vi "FPGA_SPI_ReadAuto.vi"(8 "error in (no error)":errorcluster, 9 "Bytes per Sample":u32, 10 "Samples to Read":u32) -> (0 "error out":errorcluster, 2 "Data":u8[][](array[numeric]))   [LabVIEW 2017]
uses:
  <vilib>/Utility/error.llb/Error Cluster From Error Code.vi
  <vilib>/rvi/errors/niLvFpgaAdjustHostInterfaceError.vi
  <vilib>/rvi/interface/nirviMethod/nirviMethod.xnode
  <vilib>/Rock Robotics/SystemInterfaces/System/FPGA_SystemFRC FPGA Ref.ctl
  <vilib>/FPGAPlugInAG/Dynamic/niLvFpga_ReadFifo_Dynamic.vi
  <vilib>/rvi/errors/niLvFpgaMergeErrorWithErrorCode.vi
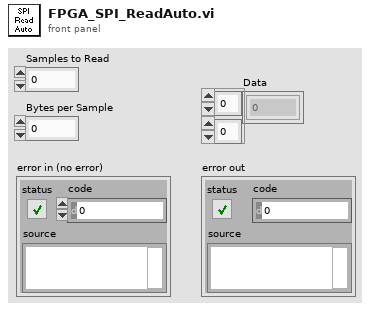
[diagram p1: front panel]
types:
  T1 = typedef "FPGA_SystemFRC FPGA Ref.ctl" = refnum<k20>
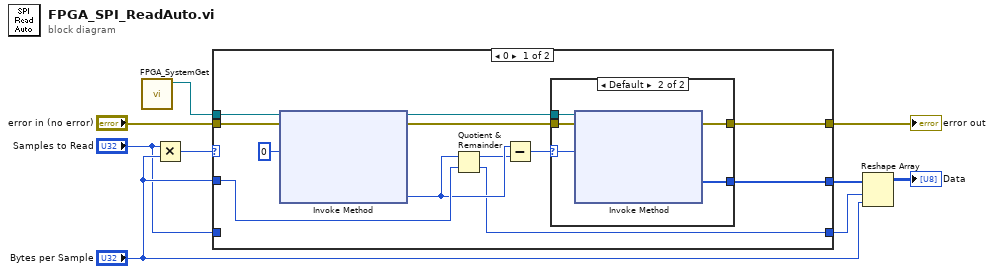
[diagram p0: block diagram]
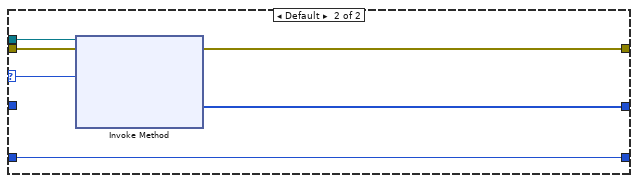
[diagram p3: hidden frame]
diagram:
  n1 = call <vilib>:"FPGA_SystemGet.vi"() -> ("FRC FPGA Ref"=w7:T1)  [unwired: 11 in]
  n2 = Multiply(x="Samples to Read", y="Bytes per Sample") -> (x*y=w5:u32)
  n3 = case shown="0" w5 {
    selector: w5 -> [_ w30]
    tunnel: [w16 w33] -> w9
    tunnel: "error in (no error)" -> [w21 w32]
    tunnel: w7 -> [w20 w31]
    tunnel: [w19 w29] -> w4
    tunnel: "Bytes per Sample" -> [w15 _]
    tunnel: [w10 w28] -> w1
    tunnel: "Samples to Read" -> [_ w28]
    frame 0 {
      n4 = xnode "Invoke Method"("FPGA VI Reference In"=w20, "error in"=w21, "Number of Elements"=u32 0) -> ("FPGA VI Reference Out"=w18:T1, "error out"=w17:errorcluster, "Elements Remaining"=w14:u32)  [unwired: 1 in, 1 out]
      n5 = Quotient & Remainder(x=w14, y=w15) -> (x-y*floor(x/y)=w13:u32, floor(x/y)=w10:u32)
      n6 = Subtract(x=w14, y=w13) -> (x-y=w12:u32)
      n7 = case shown="Default" w12 {
        selector: w12 -> [_ w24]
        tunnel: [_ w23] -> w19
        tunnel: w18 -> [_ w27]
        tunnel: w17 -> [w22 w26]
        tunnel: [w22 w25] -> w16
        frame 0 {
        }
        frame Default {
          n8 = xnode "Invoke Method"("FPGA VI Reference In"=w27, "error in"=w26, "Number of Elements"=w24) -> ("error out"=w25:errorcluster, "Data"=w23:u8[])  [unwired: 1 in, 2 out]
        }
      }
    }
    frame Default {
      n9 = xnode "Invoke Method"("FPGA VI Reference In"=w31, "error in"=w32, "Number of Elements"=w30) -> ("error out"=w33:errorcluster, "Data"=w29:u8[])  [unwired: 1 in, 2 out]
    }
  }
  "error out" <- w9
  n10 = Reshape Array(w4, w1, "Bytes per Sample") -> (→"Data":u8[][])
